vi "ExposeLogNetInfo.vi"(11 "Expose Info":T1) -> ()   [LabVIEW 2017]
uses:
  Core/ExposeInfo.ctl
  C:/Code/CMCryoSysCode/Expose/COM/CSCom/CSCom/bin/Release/CSCom.dll
  COM/CSCom/CSCom/bin/Release/CSCom.dll
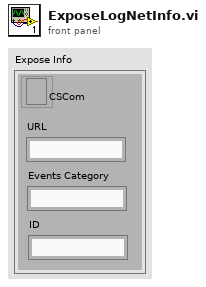
[diagram p1: front panel]
types:
  T1 = typedef "ExposeInfo.ctl" = cluster{"CSCom":refnum<k24>, "URL":string, "Events Category":string, "ID":string}
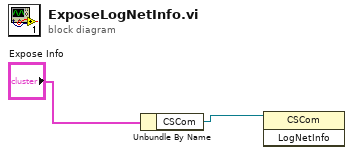
[diagram p0: block diagram]
diagram:
  n1 = Unbundle By Name("Expose Info") -> ("CSCom"=w1:refnum<k24>)
  n2 = invoke class="CSCom" method="LogNetInfo"(reference=w1) -> ()  [unwired: 2 in, 3 out]
